vi "set channel property lecroy.vi"(0 "VISA in":refnum<visa-resource-name>, 5 "Value":variant, 7 "Channel":T1={" Card.Channel"=1.12, "Crate"=0} {"Card.Channel" format="%.2f"}, 9 "Property":T2, 11 "error in":errorcluster) -> (4 "VISA out":refnum<visa-resource-name>, 15 "error out":errorcluster)   [LabVIEW 2018]
uses:
  Channel Properties.ctl
  channel.ctl
  CAEN globals.vi
  <vilib>/regexp/Match Regular Expression.xnode
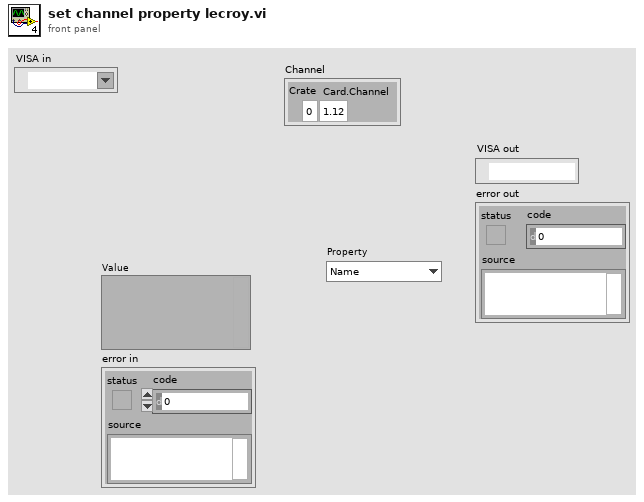
[diagram p1: front panel]
types:
  T1 = typedef "channel.ctl" = cluster{" Card.Channel":dbl, "Crate":i32}
  T2 = typedef "Channel Properties.ctl" = enum16{"Name", "Vset", "Vfile", "Vswmax", "Iset", "Enable", "Flag", "Vbackup"}
  T3 = typedef "channel_cluster.ctl" = cluster{"Channel Name":string, "Crate":i32, "Card Type":string, "Card":i32, "Channel":i32, "Status Icon":picture, "Vmon (V)":dbl, "Vset (V)":dbl, "Imon (A)":dbl, "Iset (A)":dbl, "Timestamp":string, "ON/OFF":bool, "Status":string, "Vswmax (V)":dbl, "Flag":bool, "Vfile (V)":dbl, "Error Logged":bool[], "enable_file":bool}
  T4 = enum16{"Monitor", "Demand", "Backup", "All", "None"}
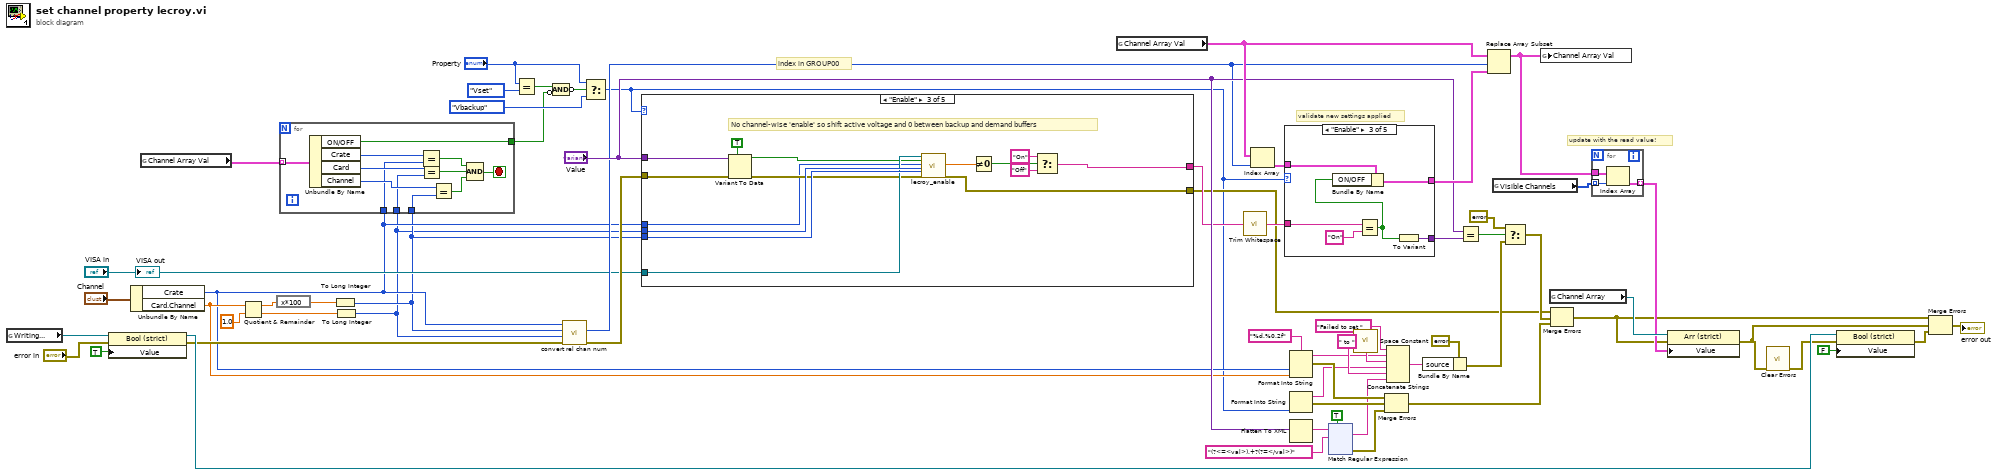
[diagram p0: block diagram]
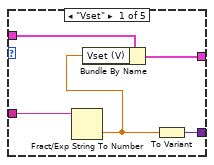
[diagram p2: hidden frame]
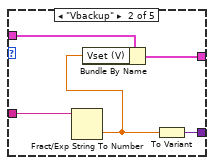
[diagram p3: hidden frame]
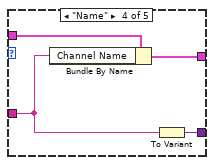
[diagram p4: hidden frame]
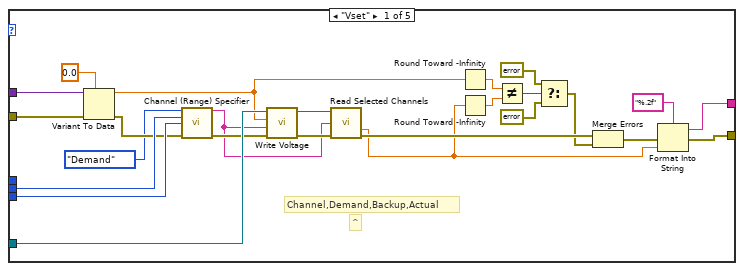
[diagram p6: hidden frame]
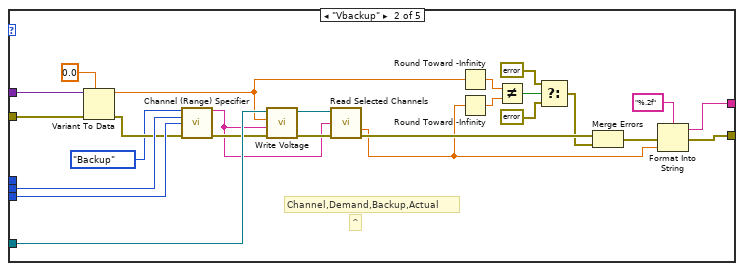
[diagram p7: hidden frame]
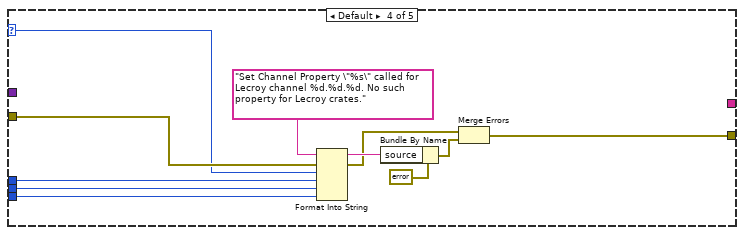
[diagram p8: hidden frame]
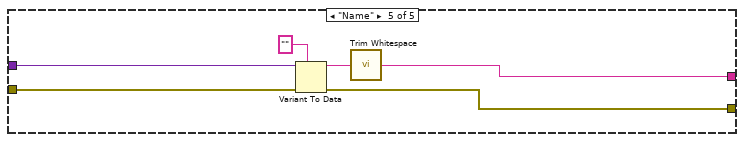
[diagram p9: hidden frame]
diagram:
  # "index in GROUP00"
  # "update with the read value!"
  # "validate new settings applied"
  n1 = global read "CAEN globals.vi" "Writing..."() -> (w60:refnum<vi>)
  n2 = property class="Bool (strict)"(reference=w60, error in="error in", "Value"=TRUE) -> (reference out=w57:refnum<vi>, error out=w24:errorcluster)
  n3 = Unbundle By Name("Channel") -> ("Crate"=w14:i32, "Card.Channel"=w23:dbl)
  n4 = global read "CAEN globals.vi" "Channel Array Val"() -> (w15:T3[])
  n5 = Quotient & Remainder(x=w23, y=1.0) -> (x-y*floor(x/y)=w17:dbl, floor(x/y)=w4:dbl)
  n6 = expression code="x*100"(w17) -> (w6:dbl)
  n7 = To Long Integer(number=w6) -> (32bit integer=w5:i32)
  n8 = To Long Integer(number=w4) -> (32bit integer=w3:i32)
  n9 = for {
    tunnel: w15 -> [w75] mode=indexing
    tunnel: w14 -> [w71]
    tunnel: w3 -> [w66]
    tunnel: w5 -> [w65]
    tunnel: [w64] -> w7
    stop <- w67 stop-if-true
    n10 = Unbundle By Name(w75) -> ("ON/OFF"=w64:bool, "Crate"=w74:i32, "Card"=w73:i32, "Channel"=w72:i32)
    n11 = Equal?(x=w74, y=w71) -> (x = y?=w69:bool)
    n12 = Equal?(x=w73, y=w66) -> (x = y?=w70:bool)
    n13 = Equal?(x=w72, y=w65) -> (x = y?=w68:bool)
    n14 = Compound Arithmetic op=AND(w69, w70, w68) -> (w67:bool)
  }
  n15 = Equal?(x="Property", y=Channel_Properties."Vset" ("x")) -> (x = y?=w12:bool)
  n16 = Compound Arithmetic op=AND(w12, invert w7) -> (invert w11:bool)
  n17 = call "convert rel chan num.vi"("error in"=w24, "Card"=w3, "Channel"=w5, "Crate"=w14) -> ("error out"=w20:errorcluster, "Absolute index"=w25:i32)  [unwired: 4 in, 2 out]
  n18 = Select(t="Property", s=w11, f=Channel_Properties."Vbackup" ("x")) -> (s? t:f=w10:T2)
  n19 = case shown="\"Enable\"" w10 {
    selector: w10 -> [_ _ _ w143 _]
    tunnel: [w87 w112 w126 _ w153] -> w22
    tunnel: "Value" -> [w99 w124 w137 _ w154]
    tunnel: [w88 w113 w131 w147 w152] -> w21
    tunnel: w20 -> [w98 w123 w134 w150 w156]
    tunnel: w14 -> [_ _ w132 w144 _]
    tunnel: "VISA in" -> [w97 w122 w138 _ _]
    tunnel: w5 -> [w95 w120 w140 w141 _]
    tunnel: w3 -> [w96 w121 w139 w142 _]
    frame "Vset" {
      # "^"
      # "Channel,Demand,Backup,Actual"
      n20 = Variant To Data(error in=w98, type=0.0 ("precision (6)"), Variant=w99) -> (data=w85:dbl, error out=w94:errorcluster)
      n21 = call "Channel (Range) Specifier.vi"("Buffer"=T4."Demand", "Card"=w96, "Channel"=w95, "error in"=w94) -> ("Channel (Range)"=w90:string, "error out"=w93:errorcluster)  [unwired: 10 in]
      n22 = call "Write Voltage.vi"("error in"=w93, "Channel+Range"=w90, "Voltage input"=w85, "VISA in"=w97) -> ("error out"=w91:errorcluster, "VISA out"=w89:refnum<visa-resource-name>)  [unwired: 5 in, 1 out]
      n23 = call "Read Selected Channels.vi"("VISA in"=w89, "C##,##DO###"=w90, "error in"=w91) -> ("First Value"=w76:dbl, "error out"=w79:errorcluster)  [unwired: 6 in, 5 out]
      n24 = Round Toward -Infinity(1:w85) -> (0:w84:dbl)
      n25 = Round Toward -Infinity(1:w76) -> (0:w83:dbl)
      n26 = Not Equal?(x=w84, y=w83) -> (x != y?=w82:bool)
      n27 = Select(t=errorcluster {"status"=TRUE, "code"=0, "source"="LeCroy Vset validation error"} ("error out"), s=w82, f=errorcluster {"status"=FALSE, "code"=0, "source"=""} ("error out")) -> (s? t:f=w78:errorcluster)
      n28 = Merge Errors(w79, w78) -> (w77:errorcluster)
      n29 = Format Into String(format string="%.2f", error in=w77, w76) -> (resulting string=w87:string, error out=w88:errorcluster)  [unwired: 1 in]
    }
    frame "Vbackup" {
      # "^"
      # "Channel,Demand,Backup,Actual"
      n30 = Variant To Data(error in=w123, type=0.0 ("precision (6)"), Variant=w124) -> (data=w110:dbl, error out=w119:errorcluster)
      n31 = call "Channel (Range) Specifier.vi"("Buffer"=T4."Backup", "Card"=w121, "Channel"=w120, "error in"=w119) -> ("Channel (Range)"=w115:string, "error out"=w118:errorcluster)  [unwired: 10 in]
      n32 = call "Write Voltage.vi"("error in"=w118, "Channel+Range"=w115, "Voltage input"=w110, "VISA in"=w122) -> ("error out"=w116:errorcluster, "VISA out"=w114:refnum<visa-resource-name>)  [unwired: 5 in, 1 out]
      n33 = call "Read Selected Channels.vi"("VISA in"=w114, "C##,##DO###"=w115, "error in"=w116) -> ("First Value"=w101:dbl, "error out"=w104:errorcluster)  [unwired: 6 in, 5 out]
      n34 = Round Toward -Infinity(1:w110) -> (0:w109:dbl)
      n35 = Round Toward -Infinity(1:w101) -> (0:w108:dbl)
      n36 = Not Equal?(x=w109, y=w108) -> (x != y?=w107:bool)
      n37 = Select(t=errorcluster {"status"=TRUE, "code"=0, "source"="LeCroy Vset validation error"} ("error out"), s=w107, f=errorcluster {"status"=FALSE, "code"=0, "source"=""} ("error out")) -> (s? t:f=w103:errorcluster)
      n38 = Merge Errors(w104, w103) -> (w102:errorcluster)
      n39 = Format Into String(format string="%.2f", error in=w102, w101) -> (resulting string=w112:string, error out=w113:errorcluster)  [unwired: 1 in]
    }
    frame "Enable" {
      # "No channel-wise 'enable' so shift active voltage and 0 between backup and demand buffers"
      n40 = Variant To Data(error in=w134, type=TRUE ("status"), Variant=w137) -> (data=w135:bool, error out=w133:errorcluster)
      n41 = call "lecroy_enable.vi"("VISA in"=w138, "Enable"=w135, "Crate"=w132, "Card"=w139, "Channel"=w140, "error in"=w133) -> ("Read Channel Voltage"=w130:dbl, "error out"=w131:errorcluster)  [unwired: 11 in, 1 out]
      n42 = Not Equal To 0?(x=w130) -> (x != 0?=w127:bool)
      n43 = Select(t="On" ("format string"), s=w127, f="Off" ("format string")) -> (s? t:f=w126:string)
    }
    frame Default {
      n44 = Format Into String(format string="Set Channel Property \"%s\" called for Lecroy channel %d.%d.%d. No such property for Lecroy crates." ("source"), error in=w150, w143, w144, w142, w141) -> (resulting string=w148:string, error out=w145:errorcluster)  [unwired: 1 in]
      n45 = Bundle By Name(cluster=errorcluster {"status"=TRUE, "code"=0, "source"=""} ("error out"), "source"=w148) -> (w146:errorcluster)
      n46 = Merge Errors(w145, w146) -> (w147:errorcluster)
    }
    frame "Name" {
      n47 = Variant To Data(error in=w156, type="" ("string"), Variant=w154) -> (data=w155:string, error out=w152:errorcluster)
      n48 = call <vilib>:"Trim Whitespace.vi"("string"=w155) -> ("trimmed string"=w153:string)  [unwired: 1 in]
    }
  }
  n49 = global read "CAEN globals.vi" "Channel Array Val"() -> (w51:T3[])
  n50 = call <vilib>:"Trim Whitespace.vi"("string"=w22) -> ("trimmed string"=w54:string)  [unwired: 1 in]
  n51 = Index Array(array=w51, index=w25) -> (element=w53:T3)
  n52 = case shown="\"Enable\"" w10 {
    tunnel: w54 -> [w161 w166 w172 w174 _]
    tunnel: [w162 w167 w173 w177 _] -> w63
    tunnel: w53 -> [w160 w165 w170 w176 w178]
    tunnel: [w158 w163 w169 w175 w178] -> w52
    frame "Vset" {
      n53 = Fract/Exp String To Number(string=w161) -> (number=w159:dbl)  [unwired: 3 in, 1 out]
      n54 = Bundle By Name(cluster=w160, "Vset (V)"=w159) -> (w158:T3)
      n55 = To Variant(anything=w159) -> (Variant=w162:variant)
    }
    frame "Vbackup" {
      n56 = Fract/Exp String To Number(string=w166) -> (number=w164:dbl)  [unwired: 3 in, 1 out]
      n57 = Bundle By Name(cluster=w165, "Vset (V)"=w164) -> (w163:T3)
      n58 = To Variant(anything=w164) -> (Variant=w167:variant)
    }
    frame "Enable" {
      n59 = Equal?(x=w172, y="On" ("x")) -> (x = y?=w168:bool)
      n60 = Bundle By Name(cluster=w170, "ON/OFF"=w168) -> (w169:T3)
      n61 = To Variant(anything=w168) -> (Variant=w173:variant)
    }
    frame "Name" {
      n62 = Bundle By Name(cluster=w176, "Channel Name"=w174) -> (w175:T3)
      n63 = To Variant(anything=w174) -> (Variant=w177:variant)
    }
    frame Default {
      # "N/A"
    }
  }
  n64 = Format Into String(format string="%d.%0.2f", w14, w23) -> (resulting string=w39:string, error out=w36:errorcluster)  [unwired: 2 in]
  n65 = Format Into String(w10) -> (resulting string=w34:string, error out=w35:errorcluster)  [unwired: 3 in]
  n66 = Flatten To XML(anything="Value") -> (xml string=w33:string)
  n67 = xnode "Match Regular Expression"("input string"=w33, "regular expression"="(?<=<val>).+?(?=</val>)" ("xml string"), "ignore case? (F)"=TRUE) -> ("whole match"=w30:string, "error out"=w29:errorcluster)  [unwired: 3 in, 3 out]
  n68 = call <vilib>:"Space Constant.vi"() -> ("String"=w43:string)
  n69 = Merge Errors(w36, w35, w29) -> (w37:errorcluster)
  n70 = Concatenate Strings("Failed to set " ("source"), w39, w43, w34, " to " ("string"), w30) -> (w45:string)
  n71 = Bundle By Name(cluster=errorcluster {"status"=TRUE, "code"=0, "source"="Value not set"} ("error in"), "source"=w45) -> (w40:errorcluster)
  n72 = Equal?(x="Value", y=w63) -> (x = y?=w62:bool)
  n73 = Replace Array Subset(array=w51, new element=w52, index=w25) -> (w50:T3[])
  n74 = global read "CAEN globals.vi" "Visible Channels"() -> (w49:i32[])
  n75 = Select(t=errorcluster {"status"=FALSE, "code"=0, "source"=""} ("error in"), s=w62, f=w40) -> (s? t:f=w61:errorcluster)
  n76 = global write "CAEN globals.vi" "Channel Array Val"(w50) -> ()
  n77 = global read "CAEN globals.vi" "Channel Array"() -> (w48:refnum<vi>)
  n78 = Merge Errors(w21, w61, w37) -> (w2:errorcluster)
  n79 = for {
    tunnel: w50 -> [w181]
    tunnel: w49 -> [w180] mode=indexing
    tunnel: [w179] -> w47 mode=indexing
    n80 = Index Array(array=w181, index=w180) -> (element=w179:T3)
  }
  n81 = property class="Arr (strict)"(reference=w48, error in=w2, "Value"=w47) -> (error out=w1:errorcluster)  [unwired: 1 out]
  n82 = call <vilib>:"Clear Errors.vi"("error in (no error)"=w1) -> ("error out"=w18:errorcluster)  [unwired: 5 in, 1 out]
  n83 = property class="Bool (strict)"(reference=w57, error in=w18, "Value"=FALSE) -> (error out=w56:errorcluster)  [unwired: 1 out]
  n84 = Merge Errors(w2, w1, w56) -> (→"error out":errorcluster)
  "VISA out" <- "VISA in"
